vi "LCM_send.vi"(8 "error in (no error)":errorcluster, 9 "DATA":string, 10 "ID":string="TEST", 11 "LCM":T1={"connection ID"=refnum, "net address"=0, "port"=7667} {"net address" format="%x"}) -> (0 "error out":errorcluster, 2 "sqenum":u32)   [LabVIEW 2015]
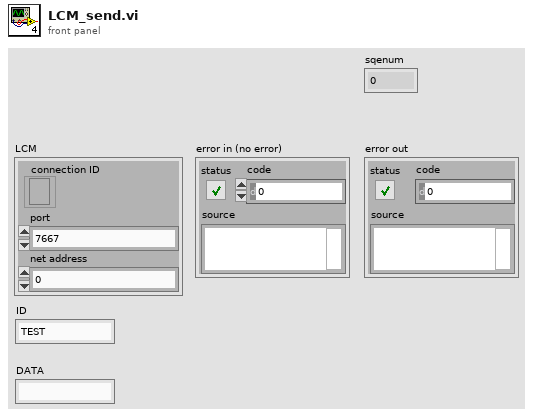
[diagram p1: front panel]
types:
  T1 = cluster{"connection ID":refnum<k16>, "net address":u32, "port":u16}
  T2 = cluster{"magic":u32, "msg_seqno":u32, "msg_size":u32, "fragment_offset":u32, "fragment_no":u16, "fragments_in_msg":u16}
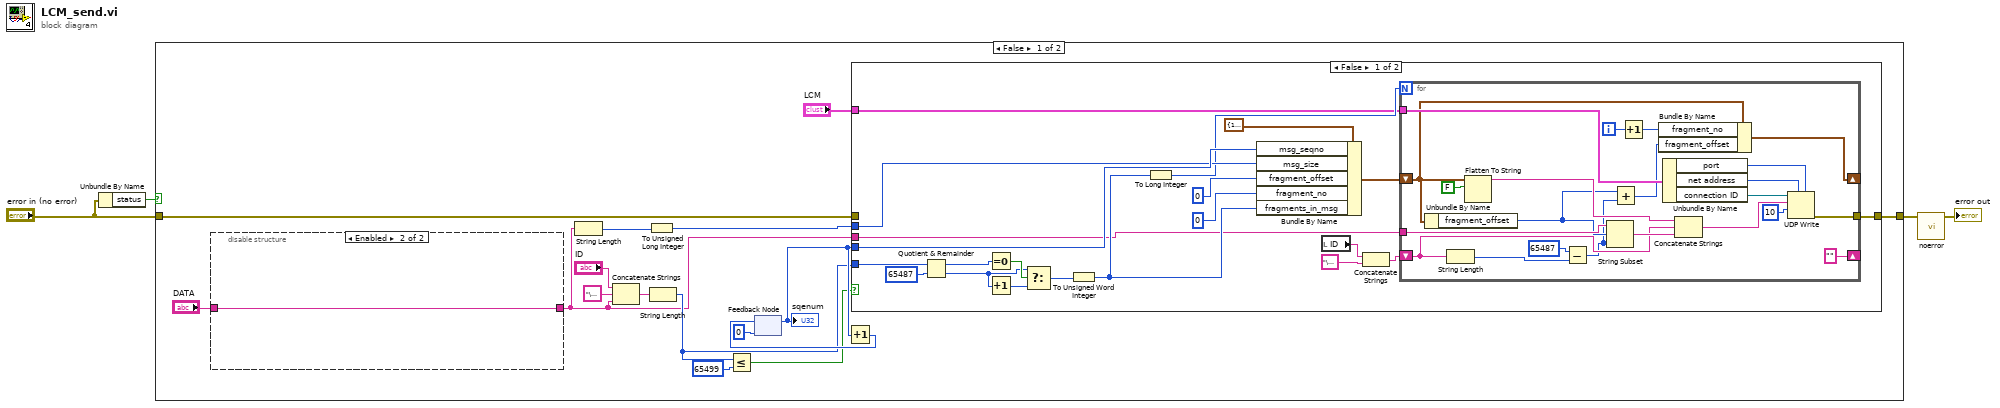
[diagram p0: block diagram]
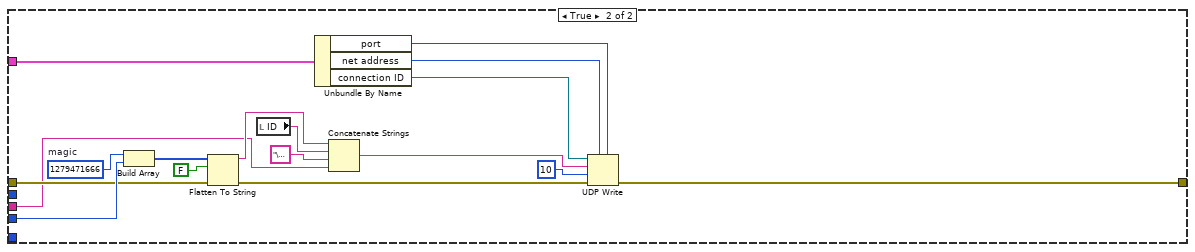
[diagram p2: hidden frame]
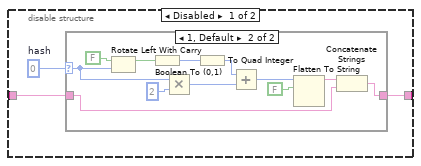
[diagram p3: hidden frame]
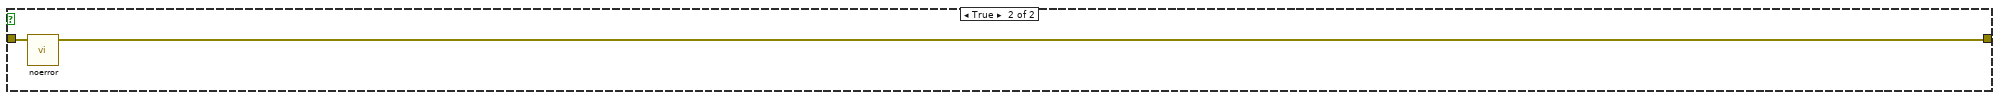
[diagram p5: hidden frame]
diagram:
  n1 = Unbundle By Name("error in (no error)") -> ("status"=w4:bool)
  n2 = case shown="False" w4 {
    tunnel: [w14 w98] -> w2
    tunnel: "error in (no error)" -> [w13 w99]
    frame False {
      n3 = disable-structure shown="Enabled" {
        disable-tunnel: "DATA" -> [w82 w97]
        disable-tunnel: [w81 w97] -> w6
        frame Disabled {
          w83 = i64 0  # hash
          n4 = case shown="1, Default" w83 {
            selector: w83 -> [_ w86]
            tunnel: w82 -> [w84 w94]
            tunnel: [w84 w93] -> w81
            frame 0 {
            }
            frame 1, Default {
              n5 = Rotate Left With Carry(2:w86, 3:FALSE ("carry")) -> (1:w90:bool)  [unwired: 1 out]
              n6 = Boolean To (0,1)(Boolean=w90) -> (0, 1=w89:i16)
              n7 = Multiply(x=w86, y=i64 2) -> (x*y=w88:i64)
              n8 = To Quad Integer(1:w89) -> (0:w87:i64)
              n9 = Add(x=w87, y=w88) -> (x+y=w85:i64)
              n10 = Flatten To String(anything=w85, prepend array or string size? (T)=FALSE) -> (data string=w95:string)  [unwired: 2 in, 2 out]
              n11 = Concatenate Strings(w95, w94) -> (w93:string)
            }
          }
        }
        frame Enabled {
        }
      }
      n12 = String Length(string=w6) -> (length=w8:i32)
      n13 = Concatenate Strings("ID", "\u0000" ("string"), w6) -> (w12:string)
      n14 = To Unsigned Long Integer(number=w8) -> (unsigned 32bit integer=w7:u32)
      n15 = String Length(string=w12) -> (length=w9:i32)
      n16 = Less Or Equal?(x=w9, y=65499 ("length (rest)")) -> (x <= y?=w10:bool)
      n17 = feedback #1(u32 0) -> (w17:u32)
      "sqenum" <- w17
      n18 = Increment(x=w17) -> (x+1=w16:u32)
      n19 = feedback-in #1(w16) -> ()
      n20 = case shown="False" w10 {
        tunnel: w17 -> [w35 w76]
        tunnel: [w21 w64] -> w14
        tunnel: w13 -> [_ w72]
        tunnel: w6 -> [w25 w69]
        tunnel: w9 -> [w41 _]
        tunnel: w7 -> [w34 _]
        tunnel: "LCM" -> [w22 w65]
        frame False {
          n21 = Quotient & Remainder(x=w41, y=65487) -> (x-y*floor(x/y)=w40:i32, floor(x/y)=w37:i32)
          n22 = Equal To 0?(x=w40) -> (x = 0?=w39:bool)
          n23 = Increment(x=w37) -> (x+1=w38:i32)
          n24 = Select(t=w37, s=w39, f=w38) -> (s? t:f=w31:i32)
          n25 = To Unsigned Word Integer(number=w31) -> (unsigned 16bit integer=w29:u16)
          n26 = To Long Integer(number=w29) -> (32bit integer=w28:i32)
          n27 = Bundle By Name(cluster=T2 {"magic"=1279471667, "msg_seqno"=1279471667, "msg_size"=1279471667, "fragment_offset"=1279471667, "fragment_no"=12339, "fragments_in_msg"=12339}, "msg_seqno"=w35, "msg_size"=w34, "fragment_offset"=u32 0, "fragment_no"=u16 0, "fragments_in_msg"=w29) -> (w23:T2)
          n28 = local read "ID"() -> (w27:string)
          n29 = Concatenate Strings(w27, "\u0000" ("string")) -> (w24:string)
          n30 = for {
            N: w28 -> [_]
            shift-right: [""] -> _
            shift-left: w24 -> [w58]
            tunnel: w25 -> [w61]
            tunnel: w22 -> [w51]
            tunnel: [w49] -> w21
            shift-right: [w46] -> _
            shift-left: w23 -> [w45]
            i -> [w48]
            n31 = Unbundle By Name(w45) -> ("fragment_offset"=w44:u32)
            n32 = String Length(string=w58) -> (length=w62:i32)
            n33 = Flatten To String(anything=w45, prepend array or string size? (T)=FALSE) -> (data string=w56:string)  [unwired: 2 in, 2 out]
            n34 = Subtract(x=65487 ("y"), y=w62) -> (x-y=w43:i32)
            n35 = String Subset(string=w61, offset (0)=w44, length (rest)=w43) -> (substring=w59:string)
            n36 = Add(x=w44, y=w43) -> (x+y=w42:u32)
            n37 = Increment(x=w48) -> (x+1=w47:i32)
            n38 = Bundle By Name(cluster=w45, "fragment_no"=w47, "fragment_offset"=w42) -> (w46:T2)
            n39 = Unbundle By Name(w51) -> ("port"=w52:u16, "net address"=w53:u32, "connection ID"=w54:refnum<k16>)
            n40 = Concatenate Strings(w56, w58, w59) -> (w50:string)
            n41 = UDP Write(address=w53, port or service name=w52, connection ID=w54, data in=w50, 9:10 ("timeout ms (25000)")) -> (error out=w49:errorcluster)  [unwired: 1 in, 1 out]
          }
        }
        frame True {
          w79 = u32 1279471666  # magic
          n42 = Build Array(w79, w76) -> (w78:u32[])
          n43 = Flatten To String(anything=w78, prepend array or string size? (T)=FALSE, error in (no error)=w72) -> (data string=w70:string, error out=w71:errorcluster)  [unwired: 1 in, 1 out]
          n44 = local read "ID"() -> (w68:string)
          n45 = Unbundle By Name(w65) -> ("port"=w73:u16, "net address"=w74:u32, "connection ID"=w75:refnum<k16>)
          n46 = Concatenate Strings(w70, w68, "\u0000" ("string"), w69) -> (w66:string)
          n47 = UDP Write(address=w74, port or service name=w73, connection ID=w75, data in=w66, 8:w71, 9:10 ("timeout ms (25000)")) -> (error out=w64:errorcluster)  [unwired: 1 out]
        }
      }
    }
    frame True {
      n48 = call "noerror.vi"("error in"=w99) -> ("error out"=w98:errorcluster)  [unwired: 10 in]
    }
  }
  n49 = call "noerror.vi"("error in"=w2) -> ("error out"=→"error out":errorcluster)  [unwired: 10 in]
